vi "数据字符串解析.vi"(7 "输入数据":string, 8 "错误输入（无错误）":errorcluster, 11 "回传数据队列":refnum<queue>) -> (0 "错误输出":errorcluster, 3 "回传数据队列":refnum<queue>)   [LabVIEW 2020]
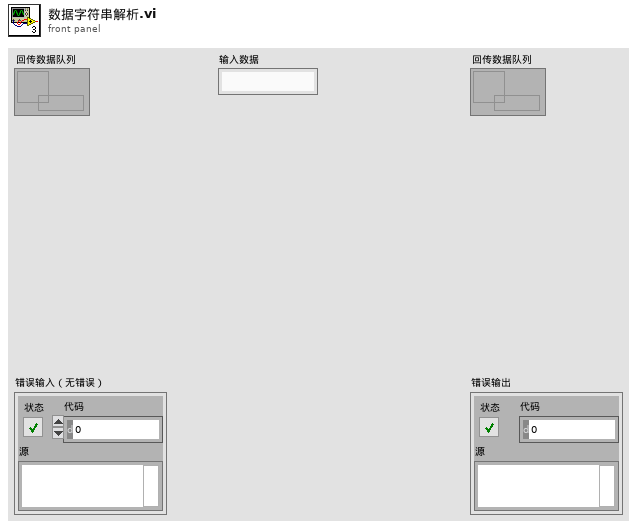
[diagram p1: front panel]
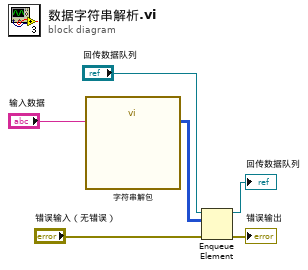
[diagram p0: block diagram]
diagram:
  n1 = call "字符串解包.vi"("data out"="输入数据") -> ("数组"=w1:i32[][])  [unwired: 10 in]
  n2 = Enqueue Element(queue="回传数据队列", element=w1, error in (no error)="错误输入（无错误）") -> (queue out=→"回传数据队列":refnum<queue>, error out=→"错误输出":errorcluster)  [unwired: 1 in, 1 out]
